vi "get Resource Directory.vi"() -> (3 "Resource Directory":path)   [LabVIEW 2021]
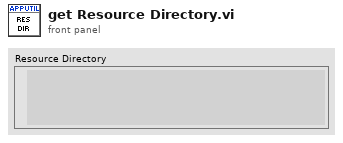
[diagram p1: front panel]
types:
  T1 = enum32{"invalid app kind", "Development System", "Run Time System", "Student Edition", "Embedded LabVIEW", "Evaluation", "Custom"}
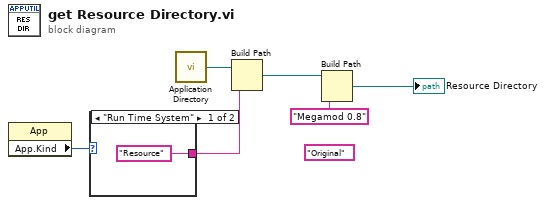
[diagram p0: block diagram]
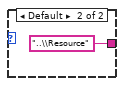
[diagram p2: hidden frame]
diagram:
  (unwired) "Original" ("name or relative path")
  n1 = property class="App"() -> ("App.Kind"=w1:T1)  [unwired: 2 in, 2 out]
  n2 = case shown="\"Run Time System\"" w1 {
    tunnel: ["Resource" ("name or relative path") "..\\Resource" ("name or relative path")] -> w5
    frame "Run Time System" {
    }
    frame Default {
    }
  }
  n3 = call <vilib>:"Application Directory.vi"() -> ("Application Directory"=w6:path)
  n4 = Build Path(base path=w6, name or relative path=w5) -> (appended path=w4:path)
  n5 = Build Path(base path=w4, name or relative path="Megamod 0.8") -> (appended path=→"Resource Directory":path)
